vi "DJGUETTA (4).vi"() -> ()   [LabVIEW 2018]
panel:
  out "discos":i32
  out "yf":i32
  out "xf":i32
  out "Discos colocados":i32[](array[numeric])
  in  "Pieza":i32(slide) scale=0.0..2.0
  out "PteVertical":i32
  out "PteHH":i32
  out "Edos":T1(ring)
  in  "Start":bool
  out "Pulsos Vertical":i32
  out "Pulsos Horizontal":i32
  in  "stop":bool
  in  "Vertical":bool
  in  "Horizontal":bool
  # "Colocados en A\n\nColocados en B\n\nColocados en C"
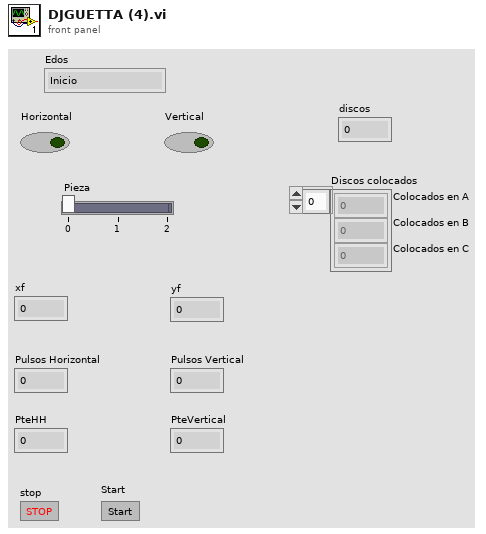
[diagram p1: front panel]
types:
  T1 = enum16{"Inicio", "Baja1", "Pausa1", "Sube1", "Pausa2", "Derecha", "Pausa3", "Baja2", "Pausa4", "Sube2", "Pausa5", "Izq", "Pausa6", "Fin"}
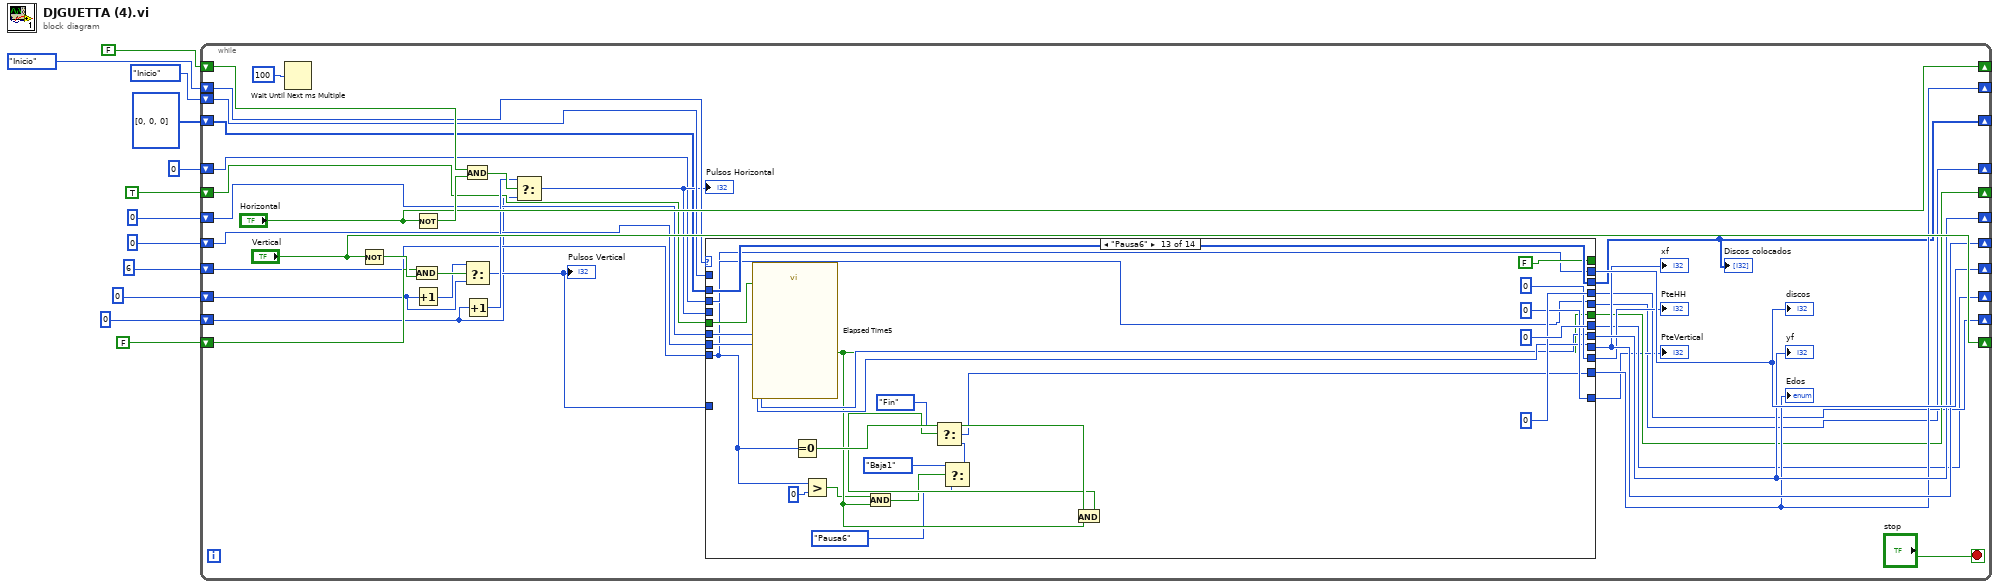
[diagram p0: block diagram]
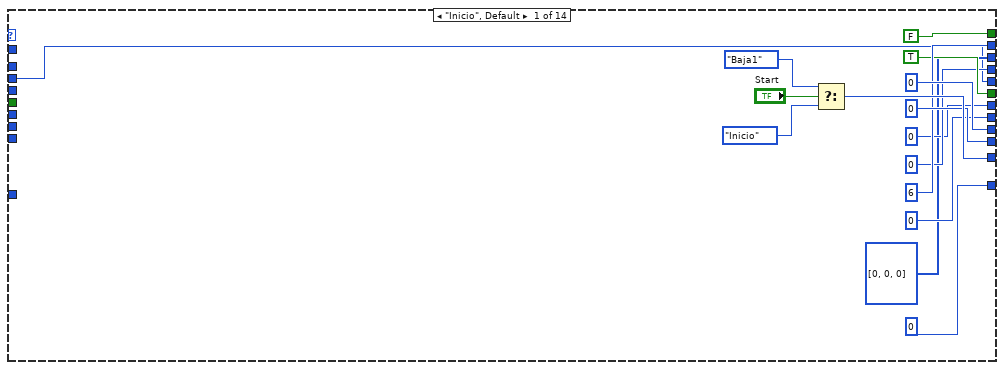
[diagram p2: hidden frame]
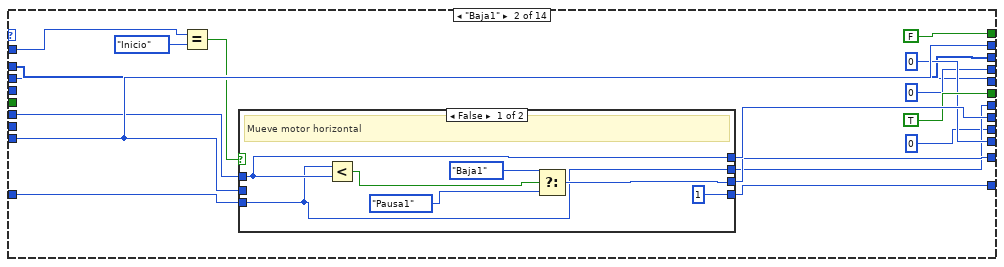
[diagram p3: hidden frame]
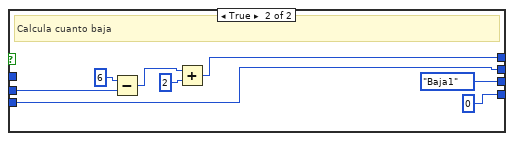
[diagram p4: hidden frame]
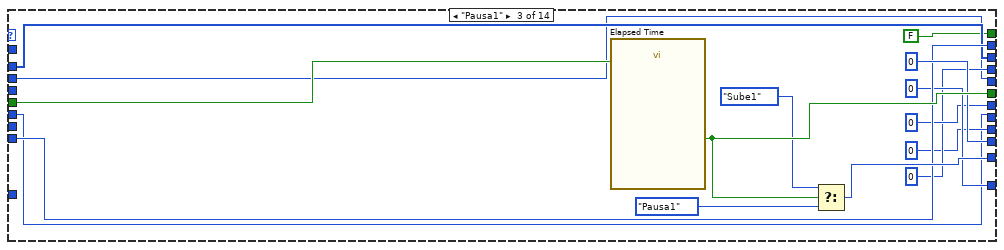
[diagram p5: hidden frame]
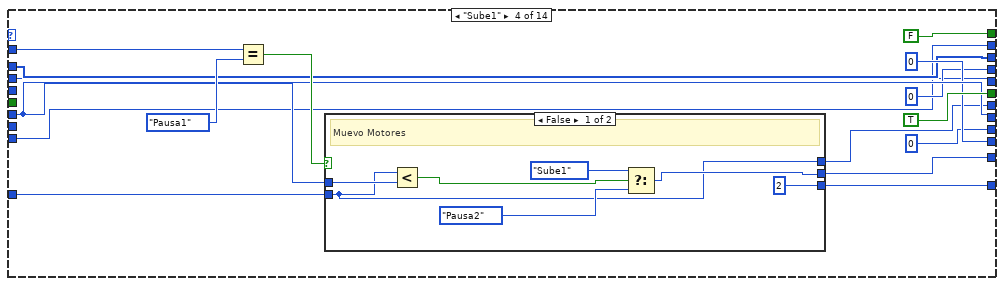
[diagram p6: hidden frame]
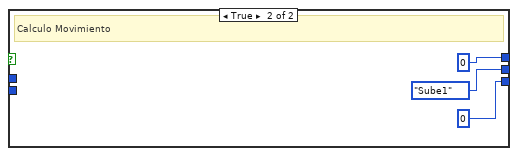
[diagram p7: hidden frame]
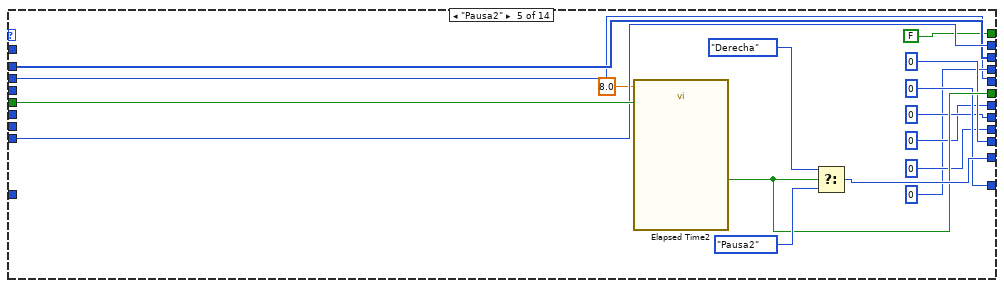
[diagram p8: hidden frame]
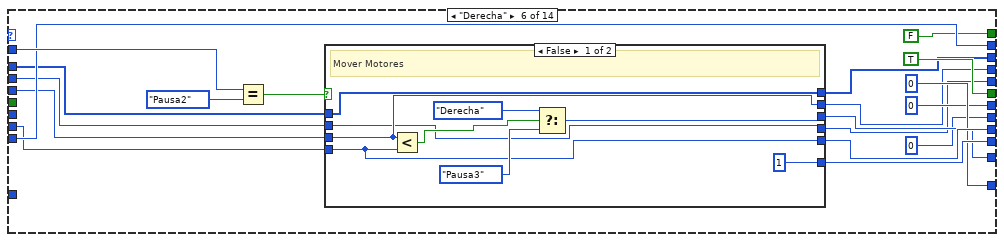
[diagram p9: hidden frame]
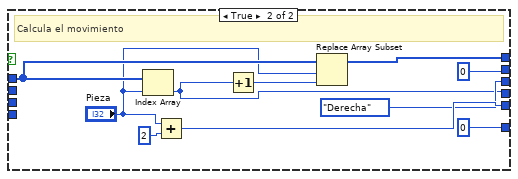
[diagram p10: hidden frame]
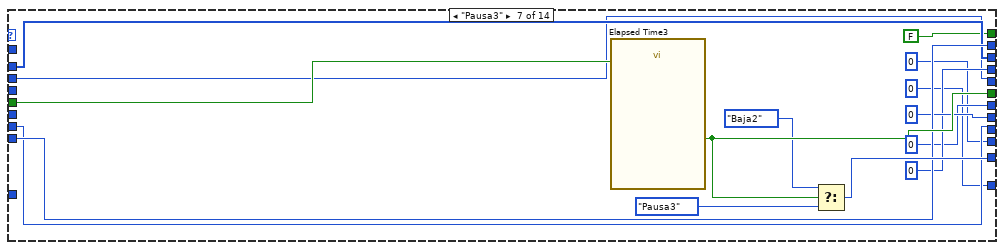
[diagram p11: hidden frame]
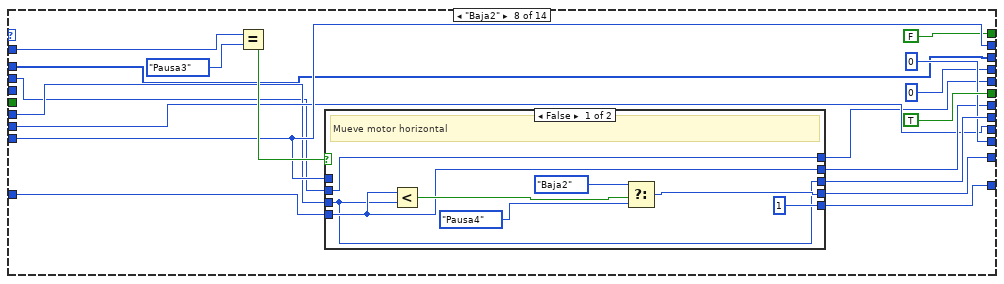
[diagram p12: hidden frame]
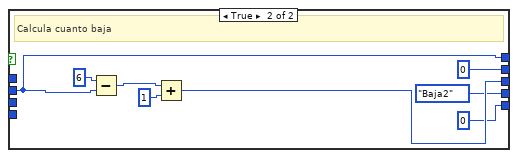
[diagram p13: hidden frame]
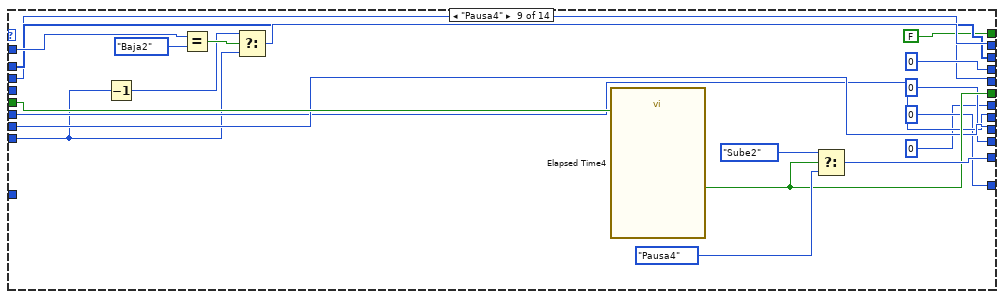
[diagram p14: hidden frame]
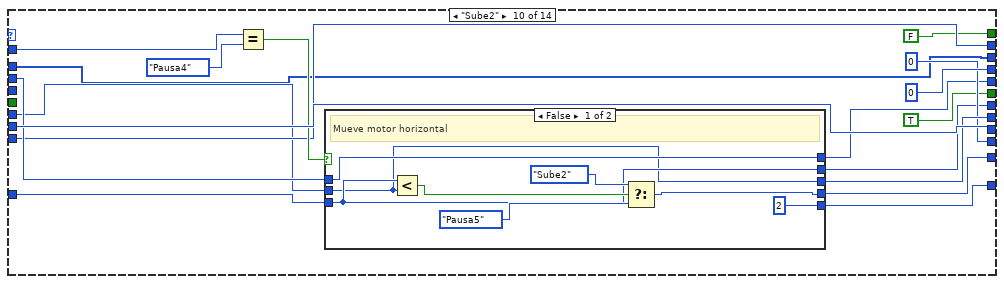
[diagram p15: hidden frame]
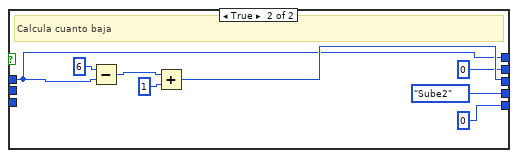
[diagram p16: hidden frame]
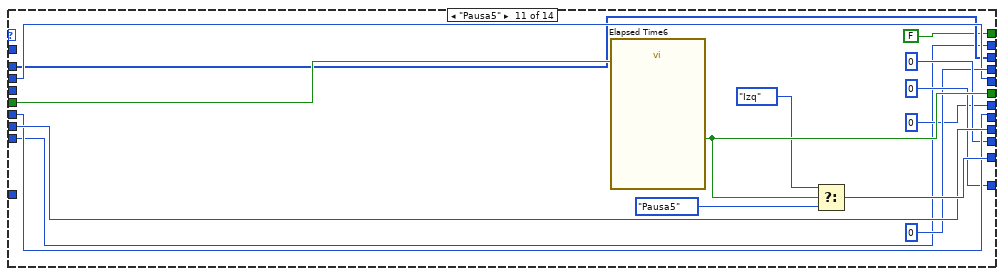
[diagram p17: hidden frame]
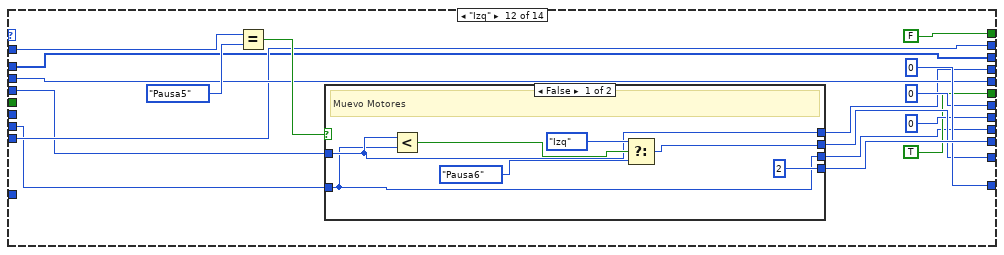
[diagram p18: hidden frame]
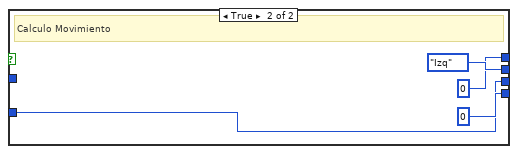
[diagram p19: hidden frame]
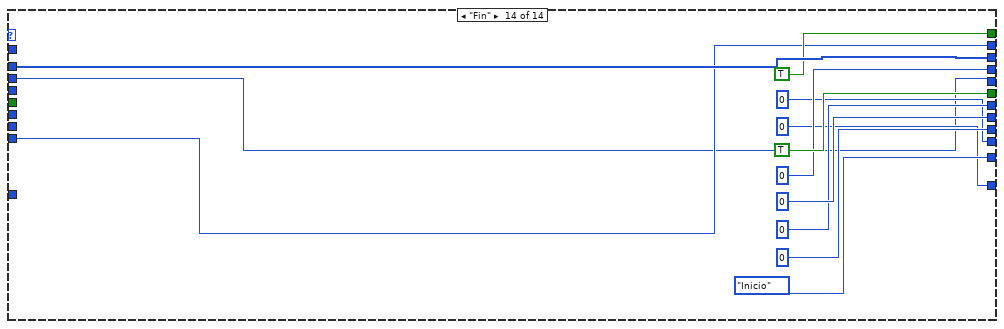
[diagram p20: hidden frame]
diagram:
  n1 = while {
    shift-right: ["Horizontal"] -> _
    shift-left: FALSE -> [w45]
    shift-right: ["Vertical"] -> _
    shift-left: FALSE -> [w43]
    shift-right: [w21] -> _
    shift-left: 0 -> [w22]
    shift-right: [w19] -> _
    shift-left: 0 -> [w36]
    shift-right: [w28] -> _
    shift-left: T1."Inicio" -> [w35]
    shift-right: [w33] -> _
    shift-left: 6 -> [w34]
    shift-right: [w29] -> _
    shift-left: 0 -> [w30]
    shift-right: [w31] -> _
    shift-left: 0 -> [w32]
    shift-left: T1."Inicio" -> [w27]
    shift-right: [w23] -> _
    shift-left: TRUE -> [w24]
    shift-right: [w16] -> _
    shift-left: i32[] [0, 0, 0] ("Discos colocados") -> [w17]
    shift-right: [w15] -> _
    shift-left: 0 -> [w14]
    stop <- "stop" stop-if-true
    n2 = Wait Until Next ms Multiple(millisecond multiple=100) -> ()  [unwired: 1 out]
    n3 = Not(x="Vertical") -> (.not. x?=w44:bool)
    n4 = And(x=w43, y=w44) -> (x .and. y?=w38:bool)
    n5 = Not(x="Horizontal") -> (.not. x?=w46:bool)
    n6 = Increment(x=w36) -> (x+1=w37:i32)
    n7 = And(x=w45, y=w46) -> (x .and. y?=w40:bool)
    n8 = Select(t=w37, s=w38, f=w36) -> (s? t:f=w26:i32)
    "Pulsos Vertical" <- w26
    n9 = Increment(x=w22) -> (x+1=w39:i32)
    n10 = Select(t=w39, s=w40, f=w22) -> (s? t:f=w20:i32)
    "Pulsos Horizontal" <- w20
    n11 = case shown="\"Pausa6\"" w35 {
      tunnel: w34 -> [_ w77 w103 w110 w144 w160 w199 w215 w243 w269 w293 w315 w344 w363]
      tunnel: [6 w77 w103 w110 w144 w160 w199 w215 w242 w269 w293 w315 w344 w363] -> w33
      tunnel: w32 -> [_ w75 w98 w119 _ _ _ w211 w252 w262 w301 _ w351 _]
      tunnel: [0 w78 w98 w119 0 0 0 w219 w252 w270 w301 0 w351 0] -> w31
      tunnel: w30 -> [_ _ _ _ _ w157 w197 w212 w253 w276 w302 w312 w352 _]
      tunnel: [0 0 0 0 0 w167 w197 w212 w253 w276 w302 w308 w352 0] -> w29
      tunnel: [w59 w76 w105 w122 w149 w164 w200 w216 w255 w267 w303 w317 w336 T1."Inicio"] -> w28
      tunnel: w27 -> [_ w68 _ w124 _ w170 _ w220 w247 w273 _ w321 _ _]
      tunnel: w26 -> [_ w74 _ w120 _ _ _ w213 _ w263 _ _ _ _]
      tunnel: [0 0 0 0 0 w166 0 0 0 0 0 w320 0 0] -> w25
      tunnel: w24 -> [_ _ w109 _ w148 _ w204 _ w258 _ w307 _ w357 _]
      tunnel: [TRUE TRUE w108 TRUE w147 TRUE w203 TRUE w254 TRUE w306 TRUE w342 TRUE] -> w23
      tunnel: [0 0 0 0 0 w161 0 0 0 0 0 w310 0 0] -> w21
      tunnel: w20 -> [_ _ _ _ _ w158 _ _ _ _ _ w311 _ _]
      tunnel: [0 w70 0 w116 0 0 0 w214 0 w264 0 0 0 0] -> w19
      tunnel: [0 w72 0 w118 0 0 0 w205 0 w271 0 0 0 0] -> w18
      tunnel: [i32[] [0, 0, 0] ("Discos colocados") w67 w97 w114 w139 w154 w192 w208 w241 w259 w295 w309 w350 w369] -> w16
      tunnel: w17 -> [_ w67 w97 w114 w139 w156 w192 w208 w241 w259 w295 w309 w350 w369]
      tunnel: [w48 w64 w95 w111 w136 w155 w190 w206 w239 w265 w296 w318 w348 w358] -> w15
      tunnel: w14 -> [w48 w64 w95 w111 w136 w152 w190 w209 w239 w272 w296 w318 w348 w358]
      tunnel: [FALSE FALSE FALSE FALSE FALSE FALSE FALSE FALSE FALSE FALSE FALSE FALSE FALSE TRUE] -> _
      frame "Inicio", Default {
        n12 = Select(t=T1."Baja1", s="Start", f=T1."Inicio") -> (s? t:f=w59:T1)
      }
      frame "Baja1" {
        n13 = Equal?(x=w68, y=T1."Inicio") -> (x = y?=w63:bool)
        n14 = case shown="False" w63 {
          tunnel: w77 -> [_ w93]
          tunnel: [w81 w90] -> w78
          tunnel: [w83 T1."Baja1" ("y")] -> w76
          tunnel: w75 -> [w81 _]
          tunnel: w74 -> [w80 w87]
          tunnel: [1 0] -> w72
          tunnel: [w80 w87] -> w70
          frame False {
            # "Mueve motor horizontal"
            n15 = Less?(x=w80, y=w81) -> (x < y?=w86:bool)
            n16 = Select(t=T1."Baja1", s=w86, f=T1."Pausa1") -> (s? t:f=w83:T1)
          }
          frame True {
            # "Calcula cuanto baja"
            n17 = Subtract(x=6, y=w93) -> (x-y=w92:i32)
            n18 = Add(x=w92, y=2) -> (x+y=w90:i32)
          }
        }
      }
      frame "Pausa1" {
        n19 = call "Elapsed Time"("Reset"=w109) -> ("Time has Elapsed"=w108:bool)  [unwired: 11 in, 7 out]
        n20 = Select(t=T1."Sube1", s=w108, f=T1."Pausa1") -> (s? t:f=w105:T1)
      }
      frame "Sube1" {
        n21 = Equal?(x=w124, y=T1."Pausa1") -> (x = y?=w125:bool)
        n22 = case shown="False" w125 {
          tunnel: [2 0] -> w118
          tunnel: [w128 T1."Sube1"] -> w122
          tunnel: [w127 0] -> w116
          tunnel: w120 -> [w127 _]
          tunnel: w119 -> [w132 _]
          frame False {
            # "Muevo Motores"
            n23 = Less?(x=w127, y=w132) -> (x < y?=w131:bool)
            n24 = Select(t=T1."Sube1", s=w131, f=T1."Pausa2") -> (s? t:f=w128:T1)
          }
          frame True {
            # "Calculo Movimiento"
          }
        }
      }
      frame "Pausa2" {
        n25 = call "Elapsed Time2"("Time Target (s)"=8.0, "Reset"=w148) -> ("Time has Elapsed"=w147:bool)  [unwired: 10 in, 7 out]
        n26 = Select(t=T1."Derecha", s=w147, f=T1."Pausa2") -> (s? t:f=w149:T1)
      }
      frame "Derecha" {
        n27 = Equal?(x=w170, y=T1."Pausa2") -> (x = y?=w168:bool)
        n28 = case shown="False" w168 {
          tunnel: [w173 w188] -> w167
          tunnel: [1 0] -> w166
          tunnel: [w176 T1."Derecha"] -> w164
          tunnel: [w175 0] -> w161
          tunnel: w158 -> [w175 _]
          tunnel: w157 -> [w173 _]
          tunnel: w156 -> [w171 w184]
          tunnel: [w172 w182] -> w155
          tunnel: [w171 w180] -> w154
          tunnel: w152 -> [w172 _]
          frame False {
            # "Mover Motores"
            n29 = Less?(x=w175, y=w173) -> (x < y?=w179:bool)
            n30 = Select(t=T1."Derecha", s=w179, f=T1."Pausa3") -> (s? t:f=w176:T1)
          }
          frame True {
            # "Calcula el movimiento"
            n31 = Index Array(array=w184, index="Pieza") -> (element=w182:i32)
            n32 = Add(x="Pieza", y=2) -> (x+y=w188:i32)
            n33 = Increment(x=w182) -> (x+1=w181:i32)
            n34 = Replace Array Subset(array=w184, new element=w181, index="Pieza") -> (w180:i32[])
          }
        }
      }
      frame "Pausa3" {
        n35 = call "Elapsed Time3"("Reset"=w204) -> ("Time has Elapsed"=w203:bool)  [unwired: 11 in, 7 out]
        n36 = Select(t=T1."Baja2", s=w203, f=T1."Pausa3") -> (s? t:f=w200:T1)
      }
      frame "Baja2" {
        n37 = Equal?(x=w220, y=T1."Pausa3") -> (x = y?=w222:bool)
        n38 = case shown="False" w222 {
          tunnel: [w224 w235] -> w219
          tunnel: [w227 T1."Baja2" ("y")] -> w216
          tunnel: [1 0] -> w205
          tunnel: w215 -> [_ _]
          tunnel: [w225 0] -> w214
          tunnel: w213 -> [w225 _]
          tunnel: w211 -> [w224 _]
          tunnel: w209 -> [w223 w231]
          tunnel: [w223 w231] -> w206
          frame False {
            # "Mueve motor horizontal"
            n39 = Less?(x=w225, y=w224) -> (x < y?=w230:bool)
            n40 = Select(t=T1."Baja2", s=w230, f=T1."Pausa4") -> (s? t:f=w227:T1)
          }
          frame True {
            # "Calcula cuanto baja"
            n41 = Subtract(x=6, y=w231) -> (x-y=w237:i32)
            n42 = Add(x=w237, y=1) -> (x+y=w235:i32)
          }
        }
      }
      frame "Pausa4" {
        n43 = Decrement(x=w243) -> (x-1=w244:i32)
        n44 = Equal?(x=w247, y=T1."Baja2") -> (x = y?=w245:bool)
        n45 = Select(t=w244, s=w245, f=w243) -> (s? t:f=w242:i32)
        n46 = call "Elapsed Time4"("Reset"=w258) -> ("Time has Elapsed"=w254:bool)  [unwired: 11 in, 7 out]
        n47 = Select(t=T1."Sube2", s=w254, f=T1."Pausa4") -> (s? t:f=w255:T1)
      }
      frame "Sube2" {
        n48 = Equal?(x=w273, y=T1."Pausa4") -> (x = y?=w275:bool)
        n49 = case shown="False" w275 {
          tunnel: [w277 w289] -> w270
          tunnel: [w281 T1."Sube2" ("y")] -> w267
          tunnel: [w279 0] -> w264
          tunnel: [2 0] -> w271
          tunnel: w272 -> [w278 w285]
          tunnel: [w278 w285] -> w265
          tunnel: w263 -> [w279 _]
          tunnel: w262 -> [w277 _]
          frame False {
            # "Mueve motor horizontal"
            n50 = Less?(x=w279, y=w277) -> (x < y?=w284:bool)
            n51 = Select(t=T1."Sube2", s=w284, f=T1."Pausa5") -> (s? t:f=w281:T1)
          }
          frame True {
            # "Calcula cuanto baja"
            n52 = Subtract(x=6, y=w285) -> (x-y=w291:i32)
            n53 = Add(x=w291, y=1) -> (x+y=w289:i32)
          }
        }
      }
      frame "Pausa5" {
        n54 = call "Elapsed Time6"("Reset"=w307) -> ("Time has Elapsed"=w306:bool)  [unwired: 11 in, 7 out]
        n55 = Select(t=T1."Izq", s=w306, f=T1."Pausa5") -> (s? t:f=w303:T1)
      }
      frame "Izq" {
        n56 = Equal?(x=w321, y=T1."Pausa5") -> (x = y?=w323:bool)
        n57 = case shown="False" w323 {
          tunnel: [w328 T1."Izq"] -> w317
          tunnel: [2 0] -> w320
          tunnel: w312 -> [w325 w332]
          tunnel: w311 -> [w326 _]
          tunnel: [w326 0] -> w310
          tunnel: [w325 w332] -> w308
          frame False {
            # "Muevo Motores"
            n58 = Less?(x=w326, y=w325) -> (x < y?=w331:bool)
            n59 = Select(t=T1."Izq", s=w331, f=T1."Pausa6") -> (s? t:f=w328:T1)
          }
          frame True {
            # "Calculo Movimiento"
          }
        }
      }
      frame "Pausa6" {
        n60 = call "Elapsed Time5"("Reset"=w357) -> ("Time has Elapsed"=w342:bool)  [unwired: 11 in, 7 out]
        n61 = Equal To 0?(x=w344) -> (x = 0?=w347:bool)
        n62 = Greater?(x=w344, y=0) -> (0:w341:bool)
        n63 = And(x=w341, y=w342) -> (x .and. y?=w340:bool)
        n64 = Select(t=T1."Baja1", s=w340, f=T1."Pausa6") -> (s? t:f=w337:T1)
        n65 = And(x=w347, y=w342) -> (x .and. y?=w346:bool)
        n66 = Select(t=T1."Fin", s=w346, f=w337) -> (s? t:f=w336:T1)
      }
      frame "Fin" {
      }
    }
    "Edos" <- w28
    "PteHH" <- w25
    "PteVertical" <- w18
    "Discos colocados" <- w16
    "xf" <- w29
    "yf" <- w31
    "discos" <- w33
  }
